vi "查找第一个标签.vi"(0 "XML String In":string caption="XML字符串输入", 11 "offset (0)":i32 caption="偏移量(0)", 12 "error in (no error)":errorcluster caption="错误输入（无错误）") -> (1 "node name":string caption="节点名", 2 "xml node attribute out":string[][](array[string]) caption="xml 节点属性", 3 "element name":string caption="元素名", 4 "before tag":string caption="标识符之前", 6 "tag":string caption="标识符", 10 "after tag":string caption="标识符之后", 13 "error out":errorcluster caption="错误输出", 14 "case":enum16{"Start Tag", "Empty Element", "Content"}(ring) caption="分支", 15 "offset past match":i32 caption="匹配后偏移量")   [LabVIEW 2017]
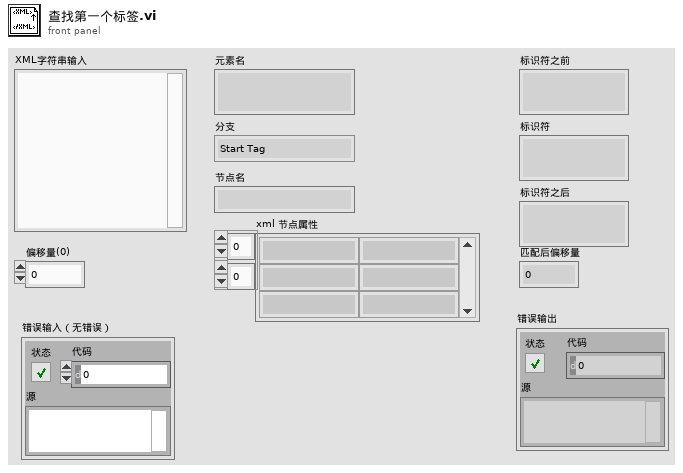
[diagram p1: front panel]
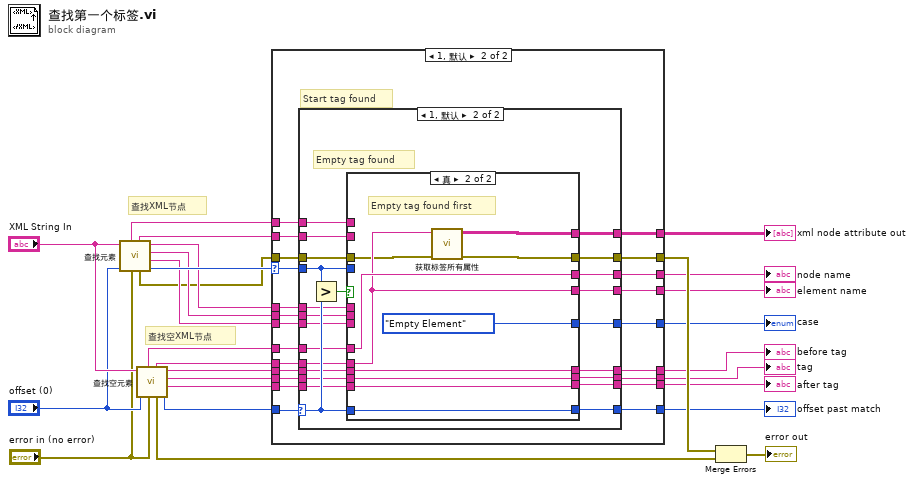
[diagram p0: block diagram]
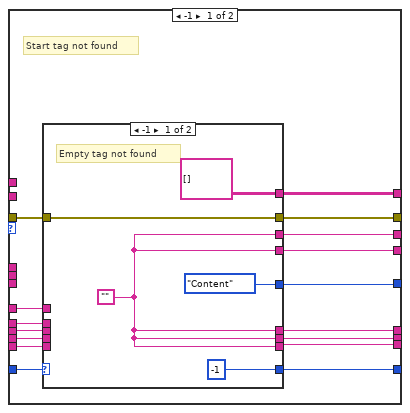
[diagram p2: hidden frame]
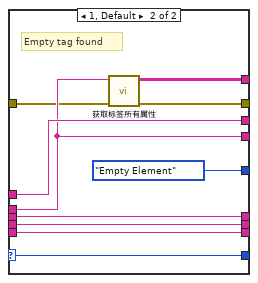
[diagram p3: hidden frame]
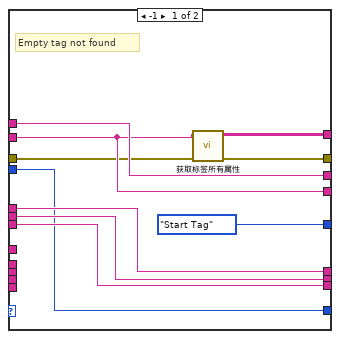
[diagram p4: hidden frame]
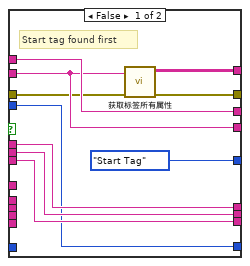
[diagram p5: hidden frame]
diagram:
  # "查找空XML节点"
  # "查找XML节点"
  n1 = call "查找元素.vi"("error in (no error)"="error in (no error)", "offset (0)"="offset (0)", "XML String In"="XML String In") -> ("offset past match"=w24:i32, "after  tag"=w21:string, "tag"=w22:string, "before tag"=w23:string, "error out"=w1:errorcluster, "element name"=w14:string, "节点名"=w5:string)  [unwired: 2 in]
  n2 = call "查找空元素.vi"("error in (no error)"="error in (no error)", "offset (0)"="offset (0)", "XML String In"="XML String In") -> ("offset past match"=w19:i32, "after  tag"=w16:string, "tag"=w17:string, "before tag"=w18:string, "error out"=w6:errorcluster, "element name"=w15:string, "node name"=w4:string)  [unwired: 2 in]
  n3 = case shown="1, 默认" w24 {
    selector: w24 -> [_ w78]
    tunnel: [w42 w80] -> w9
    tunnel: w19 -> [w43 w79]
    tunnel: w18 -> [w41 w74]
    tunnel: w17 -> [w40 w73]
    tunnel: w16 -> [w39 w72]
    tunnel: w23 -> [_ w77]
    tunnel: w22 -> [_ w76]
    tunnel: w21 -> [_ w75]
    tunnel: [w38 w71] -> w26
    tunnel: [w37 w70] -> w13
    tunnel: [w36 w69] -> w25
    tunnel: w15 -> [w34 w68]
    tunnel: w14 -> [_ w67]
    tunnel: [w35 w66] -> w12
    tunnel: [w33 w65] -> w10
    tunnel: w5 -> [_ w64]
    tunnel: w4 -> [w31 w63]
    tunnel: [w32 w62] -> w3
    tunnel: [w30 w61] -> w2
    tunnel: w1 -> [w28 w60]
    tunnel: [w29 w59] -> w27
    frame -1 {
      # "Start tag not found"
      n4 = case shown="-1" w43 {
        selector: w43 -> [_ w55]
        tunnel: [enum16{"Start Tag", "Empty Element", "Content"}."Content" enum16{"Start Tag", "Empty Element", "Content"}."Empty Element"] -> w42
        tunnel: w41 -> [_ w58]
        tunnel: w40 -> [_ w57]
        tunnel: w39 -> [_ w56]
        tunnel: [w46 w58] -> w38
        tunnel: [w46 w57] -> w37
        tunnel: [w46 w56] -> w36
        tunnel: [w46 w52] -> w35
        tunnel: w34 -> [_ w52]
        tunnel: [-1 ("offset past match") w55] -> w33
        tunnel: [w46 w53] -> w32
        tunnel: w31 -> [_ w53]
        tunnel: [string[][] [] w51] -> w30
        tunnel: [w44 w50] -> w29
        tunnel: w28 -> [w44 w49]
        frame -1 {
          w46 = ""
          # "Empty tag not found"
        }
        frame 1, Default {
          # "Empty tag found"
          n5 = call "获取标签所有属性.vi"("error in (no error)"=w49, "XML Node String In"=w52) -> ("error out"=w50:errorcluster, "xml attribute out"=w51:string[][])  [unwired: 7 in, 1 out]
        }
      }
    }
    frame 1, Default {
      # "Start tag found"
      n6 = case shown="1, 默认" w79 {
        selector: w79 -> [_ w110]
        tunnel: [enum16{"Start Tag", "Empty Element", "Content"}."Start Tag" w113] -> w80
        tunnel: w78 -> [w87 w111]
        tunnel: w77 -> [w90 w109]
        tunnel: w76 -> [w89 w108]
        tunnel: w75 -> [w88 w107]
        tunnel: w74 -> [_ w106]
        tunnel: w73 -> [_ w105]
        tunnel: w72 -> [_ w104]
        tunnel: [w90 w103] -> w71
        tunnel: [w89 w102] -> w70
        tunnel: [w88 w101] -> w69
        tunnel: w68 -> [_ w100]
        tunnel: w67 -> [w83 w98]
        tunnel: [w83 w99] -> w66
        tunnel: [w87 w97] -> w65
        tunnel: w64 -> [w85 w96]
        tunnel: w63 -> [_ w95]
        tunnel: [w85 w94] -> w62
        tunnel: [w84 w93] -> w61
        tunnel: w60 -> [w82 w92]
        tunnel: [w81 w91] -> w59
        frame -1 {
          # "Empty tag not found"
          n7 = call "获取标签所有属性.vi"("error in (no error)"=w82, "XML Node String In"=w83) -> ("error out"=w81:errorcluster, "xml attribute out"=w84:string[][])  [unwired: 7 in, 1 out]
        }
        frame 1, Default {
          # "Empty tag found"
          n8 = Greater?(x=w111, y=w110) -> (0:w112:bool)
          n9 = case shown="真" w112 {
            tunnel: [enum16{"Start Tag", "Empty Element", "Content"}."Start Tag" enum16{"Start Tag", "Empty Element", "Content"}."Empty Element"] -> w113
            tunnel: w111 -> [w120 _]
            tunnel: w110 -> [_ w130]
            tunnel: w109 -> [w123 _]
            tunnel: w108 -> [w122 _]
            tunnel: w107 -> [w121 _]
            tunnel: w106 -> [_ w133]
            tunnel: w105 -> [_ w132]
            tunnel: w104 -> [_ w131]
            tunnel: [w123 w133] -> w103
            tunnel: [w122 w132] -> w102
            tunnel: [w121 w131] -> w101
            tunnel: w100 -> [_ w126]
            tunnel: [w116 w126] -> w99
            tunnel: w98 -> [w116 _]
            tunnel: [w120 w130] -> w97
            tunnel: w96 -> [w118 _]
            tunnel: w95 -> [_ w128]
            tunnel: [w118 w128] -> w94
            tunnel: [w117 w127] -> w93
            tunnel: w92 -> [w115 w125]
            tunnel: [w114 w124] -> w91
            frame False {
              # "Start tag found first"
              n10 = call "获取标签所有属性.vi"("error in (no error)"=w115, "XML Node String In"=w116) -> ("error out"=w114:errorcluster, "xml attribute out"=w117:string[][])  [unwired: 7 in, 1 out]
            }
            frame True {
              # "Empty tag found first"
              n11 = call "获取标签所有属性.vi"("error in (no error)"=w125, "XML Node String In"=w126) -> ("error out"=w124:errorcluster, "xml attribute out"=w127:string[][])  [unwired: 7 in, 1 out]
            }
          }
        }
      }
    }
  }
  "tag" <- w13
  "before tag" <- w26
  "after tag" <- w25
  "element name" <- w12
  "offset past match" <- w10
  "case" <- w9
  "node name" <- w3
  "xml node attribute out" <- w2
  n12 = Merge Errors(w27, w6) -> (→"error out":errorcluster)
